vi "Test CRITICAL-Logger.vi"(8 "error in":errorcluster) -> (0 "error out":errorcluster)   [LabVIEW 2016, in "UT_Helper.lvlib"]
doc: "Test correct function of the Critical-Logger."
uses:
  UT_Helper.lvlib
  Source/HSE-Logger/LogLevel.ctl
  Source/HSE-Logger/LogRecord/LogRecord.lvclass/LogRecord.ctl
  Source/HSE-Logger/Handler/UserEventHandler/UserEventHandler.lvclass
  C:/Users/admin/_Git/hse-logger/Source/HSE-Logger/Handler/Handler.lvclass
  <vilib>/addons/_JKI Toolkits/Caraya/classes/Test/Test.lvclass
  Source/HSE-Logger/hse-logger.lvlib
  Source/HSE-Logger/LogRecord/LogRecord.lvclass
  <vilib>/addons/_JKI Toolkits/Caraya/classes/Assert/Assert.lvclass
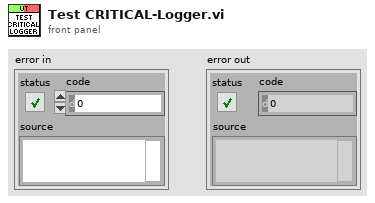
[diagram p1: front panel]
types:
  T1 = typedef "hse-logger.lvlib/LogLevel.ctl" = enum16{"DEBUG", "INFO", "WARNING", "ERROR", "CRITICAL"}
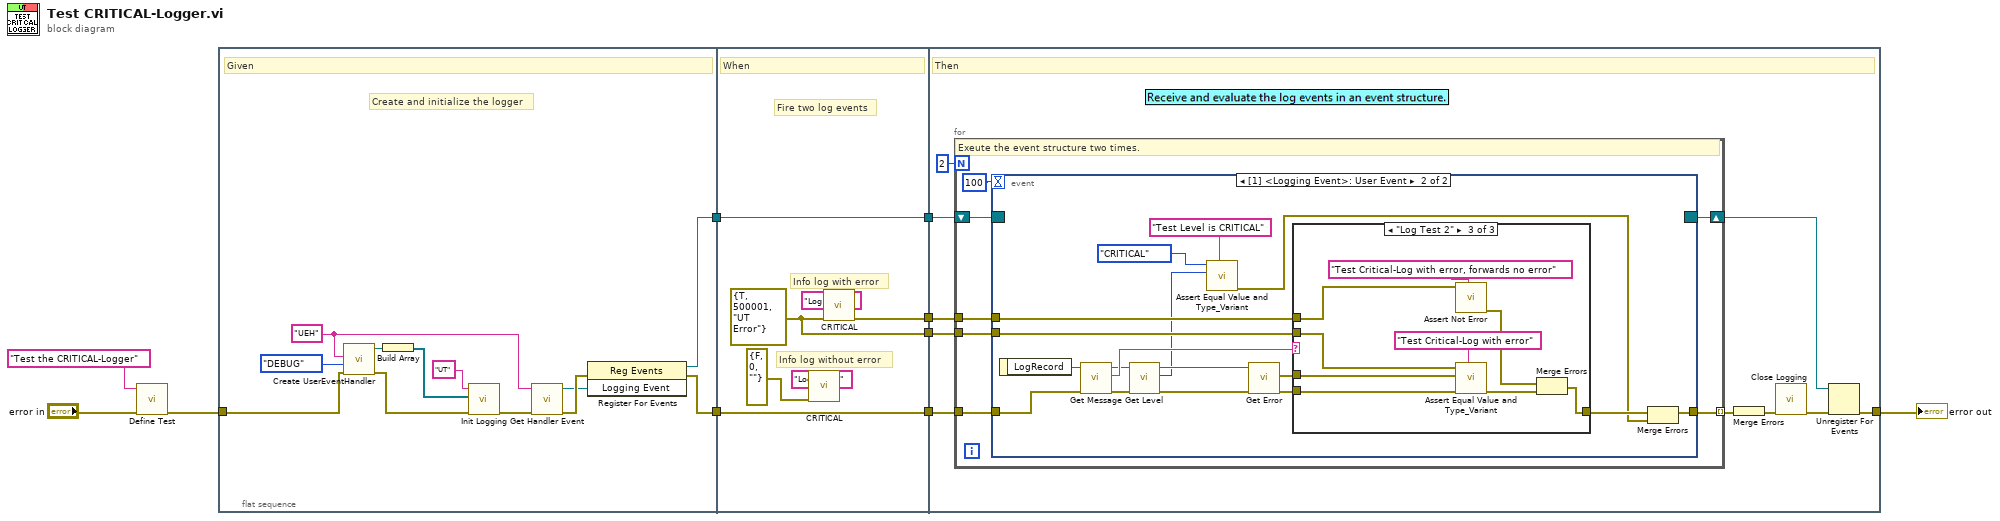
[diagram p0: block diagram]
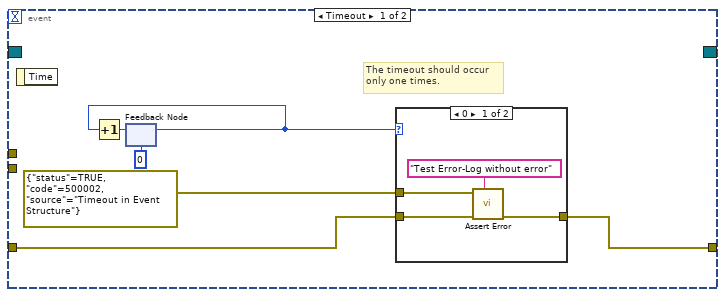
[diagram p2: hidden frame]
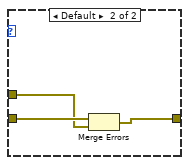
[diagram p3: hidden frame]
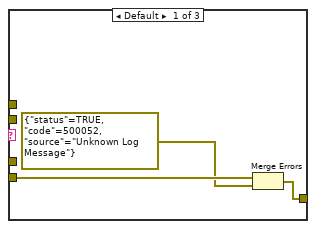
[diagram p4: hidden frame]
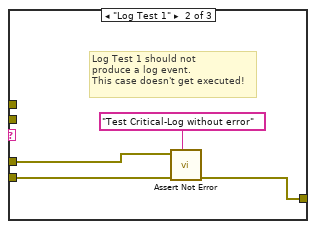
[diagram p5: hidden frame]
diagram:
  n1 = call <vilib>:"Define Test.vi"("error in (no error)"="error in", "Label (VI Title)"="Test the CRITICAL-Logger") -> ("error out"=w7:errorcluster)  [unwired: 8 in, 1 out]
  n2 = flat-sequence {
    tunnel: w7 -> [w21]
    tunnel: [w18] -> w10
    tunnel: [w13] -> w2
    tunnel: w10 -> [w29]
    tunnel: [w29] -> w6
    tunnel: w2 -> [w26]
    tunnel: [w26] -> w1
    tunnel: [w28] -> w5
    tunnel: [w27] -> w4
    tunnel: [w36] -> w9
    tunnel: w6 -> [w39]
    tunnel: w1 -> [w33]
    tunnel: w5 -> [w38]
    tunnel: w4 -> [w34]
    frame #0 {
      w12 = "UEH" ("Name")
      # "Create and initialize the logger"
      # "Given"
      n3 = call "Create UserEventHandler.vi"("error in"=w21, "Level"=LogLevel."DEBUG", "Name"=w12) -> ("error out"=w20:errorcluster, "UserEventHandler out"=w17:refnum<class "UserEventHandler.lvclass">)  [unwired: 7 in]
      n4 = Build Array(w17) -> (w16:refnum<class "UserEventHandler.lvclass">[])
      n5 = call "Init Logging.vi"("error in"=w20, "Handlers"=w16, "Name"="UT") -> ("error out"=w19:errorcluster)  [unwired: 8 in]
      n6 = call "Get Handler Event.vi"("error in"=w19, "Name"=w12) -> ("error out"=w22:errorcluster, "Logging Event"=w14:refnum<user-event>)  [unwired: 8 in]
      n7 = register-events(error in=w22, w14) -> (reference out=w13:refnum<event-registration>, error out=w18:errorcluster)  [unwired: 1 in]
    }
    frame #1 {
      w27 = errorcluster {"status"=TRUE, "code"=500001, "source"="UT Error"} ("error in")
      # "Fire two log events"
      # "Info log with error"
      # "Info log without error"
      # "When"
      n8 = call "CRITICAL.vi"("Message"="Log Test 1", "error in"=errorcluster {"status"=FALSE, "code"=0, "source"=""}) -> ()  [unwired: 9 in, 1 out]
      n9 = call "CRITICAL.vi"("Message"="Log Test 2", "error in"=w27) -> ("error out"=w28:errorcluster)  [unwired: 9 in]
    }
    frame #2 {
      # "Then"
      n10 = for {
        N: 2 -> [_]
        tunnel: w38 -> [w44]
        shift-right: [w40] -> w30
        shift-left: w33 -> [w42]
        tunnel: w39 -> [w46]
        tunnel: [w45] -> w31 mode=indexing
        tunnel: w34 -> [w43]
        # "Exeute the event structure two times."
        n11 = event shown="[1] <Logging Event>: User Event" {
          selector: w42 -> [_ _]
          dyn-events: [_ _] -> w40
          timeout: 100 -> [_ _]
          tunnel: w46 -> [w52 w76]
          tunnel: [w51 w68] -> w45
          tunnel: w44 -> [_ w72]
          tunnel: w43 -> [_ w71]
          event Timeout {
            # "The timeout should occur\nonly one times."
            n12 = event-data() -> ()  [unwired: 1 in, 1 out]
            n13 = feedback #1(0) -> (w48:i32)
            n14 = Increment(x=w48) -> (x+1=w47:i32)
            n15 = feedback-in #1(w47) -> ()
            n16 = case shown="0" w48 {
              tunnel: w52 -> [w56 w59]
              tunnel: [w55 w57] -> w51
              tunnel: errorcluster {"status"=TRUE, "code"=500002, "source"="Timeout in Event Structure"} ("error out") -> [w54 w58]
              frame 0 {
                n17 = call <vilib>:"Assert Error.vi"("Label"="Test Error-Log without error", "error in (no error)"=w56, "Error?"=w54) -> ("error out"=w55:errorcluster)  [unwired: 7 in, 1 out]
              }
              frame Default {
                n18 = Merge Errors(w59, w58) -> (w57:errorcluster)
              }
            }
          }
          event User Event {
            n19 = event-data() -> ("LogRecord"=w66:refnum<class "LogRecord.lvclass">)  [unwired: 1 in]
            n20 = call "Get Message.vi"("error in"=w76, "LogRecord in"=w66) -> ("error out"=w70:errorcluster, "Message"=w65:string, "LogRecord out"=w64:refnum<class "LogRecord.lvclass">)  [unwired: 7 in]
            n21 = call "Get Level.vi"("error in"=w70, "LogRecord in"=w64) -> ("error out"=w69:errorcluster, "Level"=w61:T1, "LogRecord out"=w63:refnum<class "LogRecord.lvclass">)  [unwired: 7 in]
            n22 = call <vilib>:"Assert Equal Value and Type_Variant.vi"("Label"="Test Level is CRITICAL", "Y"=w61, "X"=LogLevel."CRITICAL" ("Level")) -> ("error out"=w67:errorcluster)  [unwired: 7 in, 1 out]
            n23 = call "Get Error.vi"("error in"=w69, "LogRecord in"=w63) -> ("error out"=w74:errorcluster, "Error"=w75:errorcluster)  [unwired: 7 in, 1 out]
            n24 = case shown="\"Log Test 2\"" w65 {
              tunnel: w75 -> [_ w82 w90]
              tunnel: w74 -> [w79 w83 w92]
              tunnel: [w77 w81 w89] -> w73
              tunnel: w72 -> [_ _ w86]
              tunnel: w71 -> [_ _ w87]
              frame Default {
                n25 = Merge Errors(w79, errorcluster {"status"=TRUE, "code"=500052, "source"="Unknown Log Message"} ("error out")) -> (w77:errorcluster)
              }
              frame "Log Test 1" {
                # "Log Test 1 should not\nproduce a log event.\nThis case doesn't get executed!"
                n26 = call <vilib>:"Assert Not Error.vi"("Label"="Test Critical-Log without error", "error in (no error)"=w83, "Not Error?"=w82) -> ("error out"=w81:errorcluster)  [unwired: 7 in, 1 out]
              }
              frame "Log Test 2" {
                n27 = call <vilib>:"Assert Not Error.vi"("Label"="Test Critical-Log with error, forwards no error", "Not Error?"=w86) -> ("error out"=w88:errorcluster)  [unwired: 8 in, 1 out]
                n28 = call <vilib>:"Assert Equal Value and Type_Variant.vi"("Label"="Test Critical-Log with error", "error in (no error)"=w92, "Y"=w90, "X"=w87) -> ("error out"=w91:errorcluster)  [unwired: 6 in, 1 out]
                n29 = Merge Errors(w88, w91) -> (w89:errorcluster)
              }
            }
            n30 = Merge Errors(w73, w67) -> (w68:errorcluster)
          }
        }
      }
      n31 = Merge Errors(w31) -> (w35:errorcluster)
      n32 = call "Close Logging.vi"("error in"=w35) -> ("error out"=w37:errorcluster)  [unwired: 10 in]
      n33 = Unregister For Events(event registration refnum=w30, error in=w37) -> (error out=w36:errorcluster)
    }
  }
  "error out" <- w9
